vi "Eval y=f(x) Prep1 (VI).vi"(4 "sign":i32(ring) items=["y=f(x)", "y=-f(x)"], 6 "data":variant, 7 "f(x)":T1, 8 "error in":i32, 9 "number of points":u32, 10 "start":dbl format="%.2f", 11 "end":dbl format="%.2f") -> (0 "error out":i32, 1 "points II":dbl[](array[numeric]), 2 "points I":dbl[](array[numeric]), 3 "points":dbl[](array[numeric]), 5 "random summand":dbl format="%.2f")   [LabVIEW 2014, in "NI_Gmath.lvlib"]
uses:
  NI_Gmath.lvlib
  functionRefnum.ctl
  Ramp Pattern by Samples.vi
  NI_AALBase.lvlib
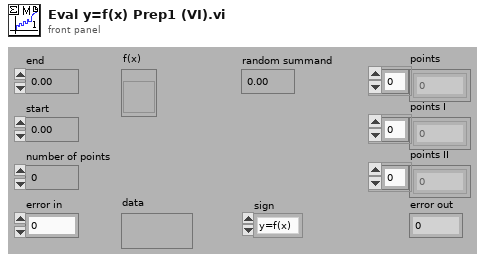
[diagram p1: front panel]
types:
  T1 = typedef "NI_Gmath.lvlib/functionRefnum.ctl" = refnum<vi>
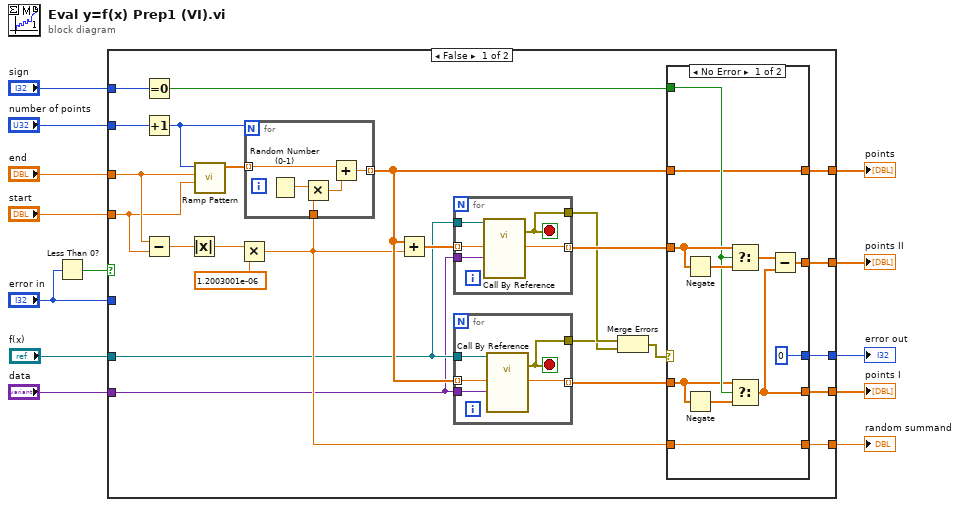
[diagram p0: block diagram]
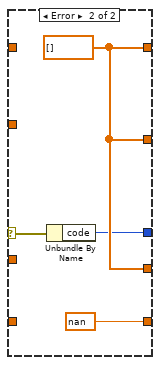
[diagram p2: hidden frame]
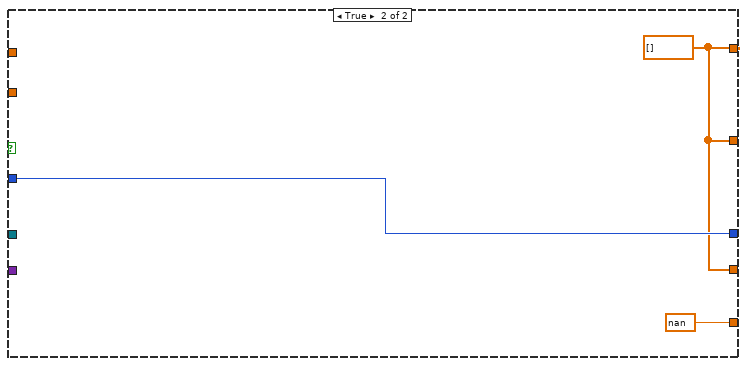
[diagram p3: hidden frame]
diagram:
  n1 = Less Than 0?(x="error in") -> (x < 0?=w13:bool)
  n2 = case shown="False" w13 {
    tunnel: "error in" -> [_ w71]
    tunnel: [w22 w71] -> w11
    tunnel: [w24 w70] -> w9
    tunnel: [w29 w70] -> w8
    tunnel: [w34 w70] -> w7
    tunnel: [w20 nan] -> w10
    tunnel: "sign" -> [w19 _]
    tunnel: "number of points" -> [w18 _]
    tunnel: "end" -> [w17 _]
    tunnel: "start" -> [w16 _]
    tunnel: "f(x)" -> [w15 _]
    tunnel: "data" -> [w14 _]
    frame False {
      n3 = Equal To 0?(x=w19) -> (x = 0?=w30:bool)
      n4 = Increment(x=w18) -> (x+1=w33:u32)
      n5 = Subtract(x=w17, y=w16) -> (x-y=w38:dbl)
      n6 = Absolute Value(x=w38) -> (abs(x)=w37:dbl)
      n7 = call-poly "Ramp Pattern.vi"("start"=w16, "end"=w17, "samples"=w33) -> ("Ramp Pattern"=w32:dbl[])  [unwired: 7 in, 1 out]
      n8 = Multiply(x=w37, y=1.2003001e-06) -> (x*y=w21:dbl)
      n9 = for {
        N: w33 -> [_]
        tunnel: [w65] -> w25 mode=indexing
        tunnel: w21 -> [w67]
        tunnel: w32 -> [w64] mode=indexing
        n10 = Random Number (0-1)() -> (number: 0 to 1=w68:dbl)
        n11 = Multiply(x=w68, y=w67) -> (x*y=w66:dbl)
        n12 = Add(x=w64, y=w66) -> (x+y=w65:dbl)
      }
      n13 = Add(x=w25, y=w21) -> (x+y=w35:dbl[])
      n14 = for {
        tunnel: w35 -> [w58] mode=indexing
        tunnel: [w55] -> w31 mode=indexing
        tunnel: w14 -> [w56]
        tunnel: w15 -> [w57]
        tunnel: [w54] -> w27
        stop <- w54 stop-if-true
        n15 = call-by-ref "?"(reference=w57, "Variant"=w56, "x"=w58) -> (error out=w54:errorcluster, "f(x)"=w55:dbl)  [unwired: 4 in, 1 out]
      }
      n16 = for {
        tunnel: w25 -> [w63] mode=indexing
        tunnel: [w60] -> w28 mode=indexing
        tunnel: w14 -> [w61]
        tunnel: w15 -> [w62]
        tunnel: [w59] -> w26
        stop <- w59 stop-if-true
        n17 = call-by-ref "?"(reference=w62, "Variant"=w61, "x"=w63) -> (error out=w59:errorcluster, "f(x)"=w60:dbl)  [unwired: 4 in, 1 out]
      }
      n18 = Merge Errors(w27, w26) -> (w23:errorcluster)
      n19 = case shown="No Error" w23 {
        selector: w23 -> [_ w52]
        tunnel: [w49 w53] -> w34
        tunnel: w31 -> [w46 _]
        tunnel: w30 -> [w45 _]
        tunnel: [w43 w53] -> w29
        tunnel: w28 -> [w42 _]
        tunnel: w25 -> [w41 _]
        tunnel: [w41 w53] -> w24
        tunnel: [0 w51] -> w22
        tunnel: w21 -> [w39 _]
        tunnel: [w39 nan] -> w20
        frame No Error {
          n20 = Negate(x=w46) -> (-x=w48:dbl[])
          n21 = Negate(x=w42) -> (-x=w47:dbl[])
          n22 = Select(t=w46, s=w45, f=w48) -> (s? t:f=w44:dbl[])
          n23 = Select(t=w42, s=w45, f=w47) -> (s? t:f=w43:dbl[])
          n24 = Subtract(x=w44, y=w43) -> (x-y=w49:dbl[])
        }
        frame Error {
          w53 = dbl[] []
          n25 = Unbundle By Name(w52) -> ("code"=w51:i32)
        }
      }
    }
    frame True {
      w70 = dbl[] []
    }
  }
  "error out" <- w11
  "random summand" <- w10
  "points" <- w9
  "points I" <- w8
  "points II" <- w7
